vi "Tick Count (ms).vi"(8 "error in (no error)":errorcluster) -> (0 "error out":errorcluster, 3 "millisecond timer value":u32)   [LabVIEW 2017]
doc: "Returns the millisecond timer value of the Tick Count (ms) primitive with error in and error out terminals added."
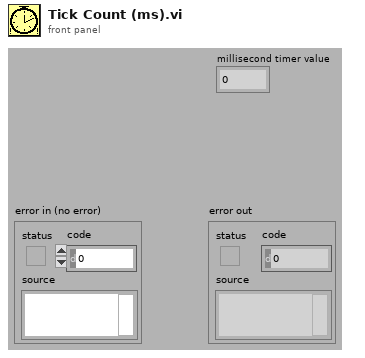
[diagram p1: front panel]
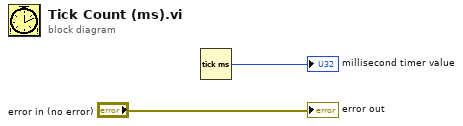
[diagram p0: block diagram]
diagram:
  n1 = Tick Count (ms)() -> (millisecond timer value=→"millisecond timer value":u32)
  "error out" <- "error in (no error)"
